vi "Initialize.vi"(6 "Schedule":string[](array[string]), 8 "error in (no error)":errorcluster, 9 "Minor Frame Time (100 us)":u32=100, 11 "ID":string) -> (0 "error out":errorcluster, 3 "Major Frame out":refnum<class "Major Frame.lvclass">)   [LabVIEW 2020, in "BCI-1553 API.lvlib" / "Major Frame.lvclass"]
doc: "Generates a Major Frame object that can be used in a Bus Controller to define a sequence of Minor Frames and Messages. The ID must be unique to this Major Frame. The Minor Frame Time dictates the amount of time from the start of one Minor Frame to the start of the next Minor Frame. The Schedule is an array of strings that defines the exact order in which to execute Minor Frame IDs and Message IDs. The Minor Frame Time is only precise to the nearest 100 us."
uses:
  Major Frame.lvclass
  Major Frame.lvclass/Major Frame.ctl
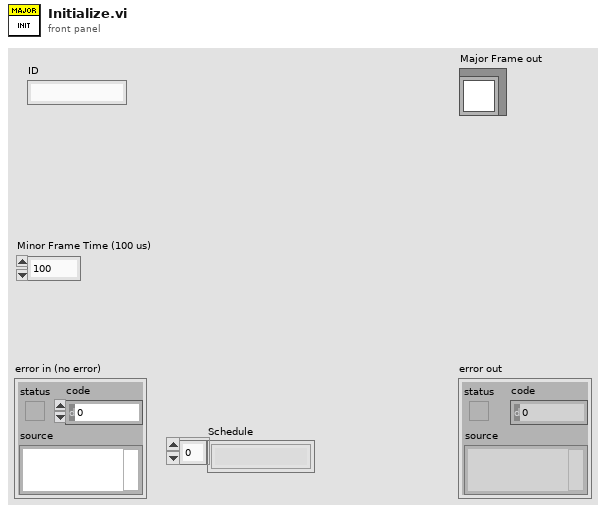
[diagram p1: front panel]
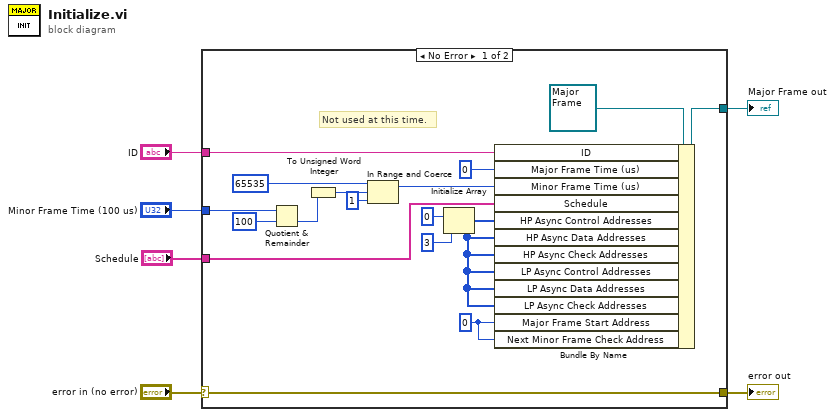
[diagram p0: block diagram]
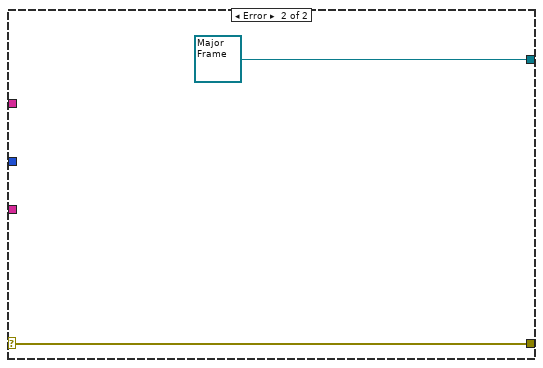
[diagram p2: hidden frame]
diagram:
  n1 = case shown="No Error" "error in (no error)" {
    selector: "error in (no error)" -> [w23 w25]
    tunnel: [w23 w25] -> w5
    tunnel: [w21 refnum<class "Major Frame.lvclass"> refnum ("Major Frame in")] -> w4
    tunnel: "ID" -> [w20 _]
    tunnel: "Minor Frame Time (100 us)" -> [w14 _]
    tunnel: "Schedule" -> [w7 _]
    frame No Error {
      w16 = u16 0 ("Major Frame Start Address")
      # "Not used at this time."
      n2 = Quotient & Remainder(x=w14, y=u32 100) -> (floor(x/y)=w13:u32)  [unwired: 1 out]
      n3 = To Unsigned Word Integer(number=w13) -> (unsigned 16bit integer=w11:u16)
      n4 = In Range and Coerce(upper limit=u16 65535, x=w11, lower limit=u16 1) -> (coerced(x)=w10:u16)  [unwired: 1 out]
      n5 = Initialize Array(u16 0 ("HP Async Control Addresses"), 3 ("dimension size")) -> (w15:u16[])
      n6 = Bundle By Name(cluster=refnum<class "Major Frame.lvclass"> refnum ("Major Frame in"), "ID"=w20, "Major Frame Time (us)"=u16 0, "Minor Frame Time (us)"=w10, "Schedule"=w7, "HP Async Control Addresses"=w15, "HP Async Data Addresses"=w15, "HP Async Check Addresses"=w15, "LP Async Control Addresses"=w15, "LP Async Data Addresses"=w15, "LP Async Check Addresses"=w15, "Major Frame Start Address"=w16, "Next Minor Frame Check Address"=w16) -> (w21:refnum<class "Major Frame.lvclass">)
    }
    frame Error {
    }
  }
  "error out" <- w5
  "Major Frame out" <- w4
